vi "Set Group Offset.vi"(10 "group offset":u64, 11 "Transfer in":refnum<class "Transfer.lvclass">) -> (3 "Transfer out":refnum<class "Transfer.lvclass">)   [LabVIEW 2017, in "Data Sharing Framework Core.lvlib" / "Data Sharing Framework Engine.lvlib" / "Transfer.lvclass"]
uses:
  Transfer.lvclass
  Transfer.lvclass/Transfer.ctl
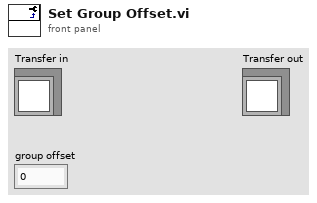
[diagram p1: front panel]
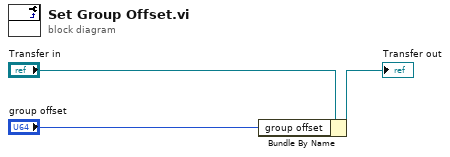
[diagram p0: block diagram]
diagram:
  n1 = Bundle By Name(cluster="Transfer in", "group offset"="group offset") -> (→"Transfer out":refnum<class "Transfer.lvclass">)
